vi "Time Elapsed.vi"(8 "error in (no error)":errorcluster, 10 "TE":i32, 11 "Reset":bool) -> (0 "error out":errorcluster, 3 "Timeout":bool)   [LabVIEW 2019, in "Zen Analytics.lvlib" / "Zen Analytics.lvclass"]
uses:
  Zen Analytics.lvclass
panel:
  out "Elapsed Time (s)":dbl
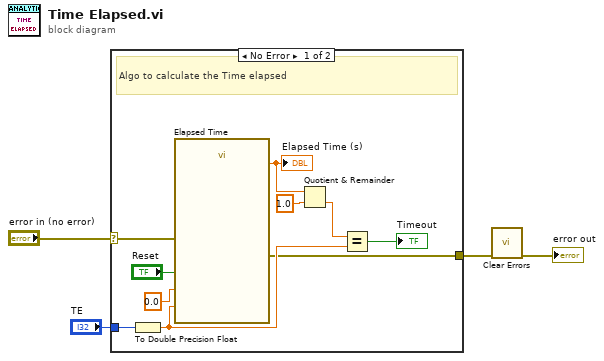
[diagram p0: block diagram]
diagram:
  n1 = case shown="No Error" "error in (no error)" {
    selector: "error in (no error)" -> [w6 w15]
    tunnel: [w5 w15] -> w2
    tunnel: "TE" -> [w9 _]
    frame No Error {
      # "Algo to calculate the Time elapsed"
      n2 = To Double Precision Float(number=w9) -> (double precision float=w8:dbl)
      n3 = call "Elapsed Time"("Time Target (s)"=w8, "Reset"="Reset", "error in (no error)"=w6, "Set Start Time (s)"=0.0) -> ("Elapsed Time (s)"=w11:dbl, "error out"=w5:errorcluster)  [unwired: 8 in, 6 out]
      "Elapsed Time (s)" <- w11
      n4 = Quotient & Remainder(x=w11, y=1.0) -> (floor(x/y)=w13:dbl)  [unwired: 1 out]
      n5 = Equal?(x=w13, y=w8) -> (x = y?=→"Timeout":bool)
    }
    frame Error {
    }
  }
  n6 = call <vilib>:"Clear Errors.vi"("error in (no error)"=w2) -> ("error out"=→"error out":errorcluster)  [unwired: 5 in, 1 out]
